vi "XNET Example IP Stack Config - Add Proxy Server.vi"(0 "config in":string, 1 "forwarding destination address":string, 2 "forwarding destination port":u16, 5 "protocol":string(combo)="tcp", 7 "direction":string(combo)="outbound", 9 "listen port":u16, 11 "error in (no error)":errorcluster, 12 "listen address":string, 13 "forwarding source address":string, 14 "forwarding source port":u16) -> (4 "config out":string, 15 "error out":errorcluster)   [LabVIEW 2018]
doc: "This example subVI adds configuration for a single proxy server instance to an existing JSON configuration string for use with XNET IP Stack Create.vi. Configuration parameter definitions:\n\nprotocol: Protocol to use for the proxy server, which can be one of 1) tcp, 2) udp.\n\ndirection: Direction to use for the proxy server, which can be one of 1) outbound, 2) inbound. When using TCP, this specifies the direction of the TCP connection. Once connected, TCP communication is always bidirectional through a single proxy server. When using UDP, this specifies the direction of communication, which is always unidirectional. Use two proxy servers if you require bidirectional UDP communication.\n\nlisten address: The proxy server listens for data on this address. This can be 'any', 'localhost', or a valid IPv4 or IPv6 address using standard IETF syntax. This property is optional; if not provided or if set to an empty string, outbound servers use the default value 'localhost', and inbound servers use the default value 'any'.\n\nlisten port: The proxy server listens for data on this port. Values from 1-65535 identify a valid port number.\n\nforwarding destination address: The proxy server forwards all received data to this address. This can be 'localhost' or a valid IPv4 or IPv6 address using standard IETF syntax.\n\nforwarding destination port: The proxy server forwards all received data to this port. Values from 1-65535 identify a valid port number.\n\nforwarding source address: The proxy server forwards all data using this source address. This can be 'any', 'localhost', or a valid IPv4 or IPv6 address using standard IETF syntax. This property is optional; if not provided or if set to an empty string, the default value 'any' is used.\n\nforwarding source port: The proxy server forwards all data using this source port. Values from 0-65535 identify a valid port number. This property is optional; if not provided, the default value 0 is used, which assigns a randomly-selected port.\n\nYou can re-use this subVI in one of two ways: a) copy the subVI from the example diagram to your VI diagram, which re-uses the subVI unchanged (located in the XNET library), or b) use Save As to create a copy of the subVI in your application folder, and change as needed."
uses:
  XNET Example IP Stack Config - Stack.ctl
  XNET Example IP Stack Config - XNET Interface.ctl
  XNET Example IP Stack Config - MAC.ctl
  XNET Example IP Stack Config - VLAN.ctl
  XNET Example IP Stack Config - Static Address.ctl
  XNET Example IP Stack Config - Static IPv6 Address.ctl
  XNET Example IP Stack Config - Proxy Server.ctl
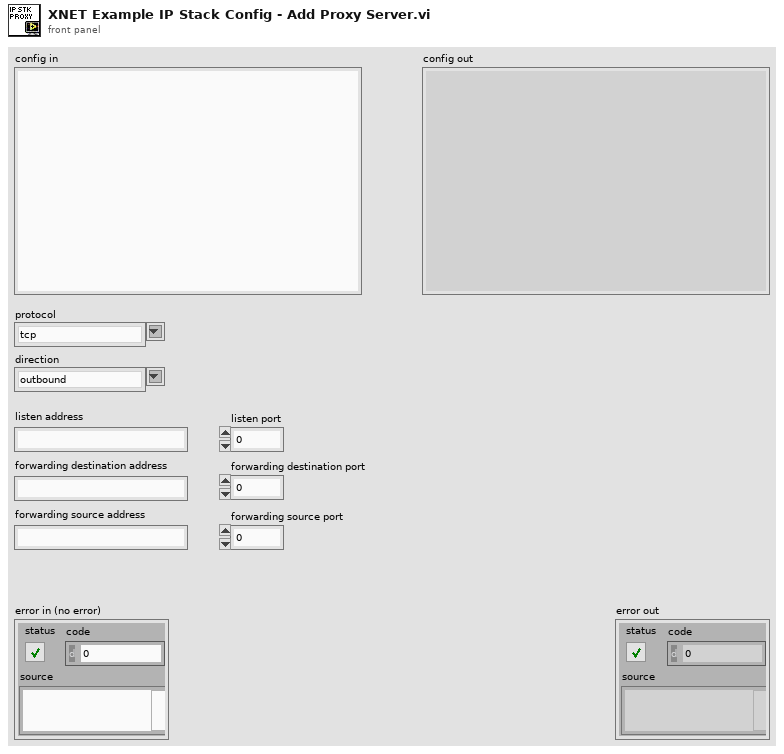
[diagram p1: front panel]
types:
  T1 = typedef "XNET Example IP Stack Config - Proxy Server.ctl" = cluster{"protocol":string, "direction":string, "listenAddress":string, "listenPort":u16, "forwardingDestinationAddress":string, "forwardingDestinationPort":u16, "forwardingSourceAddress":string, "forwardingSourcePort":u16}
  T2 = typedef "XNET Example IP Stack Config - Stack.ctl" = cluster{"schema":string, "xnetInterfaces":T3[], "proxyServers":T1[]}
  T3 = typedef "XNET Example IP Stack Config - XNET Interface.ctl" = cluster{"name":string, "MACs":T4[]}
  T4 = typedef "XNET Example IP Stack Config - MAC.ctl" = cluster{"address":string, "VLANs":T5[]}
  T5 = typedef "XNET Example IP Stack Config - VLAN.ctl" = cluster{"name":string, "isTagged":bool, "id":u16, "IPv4":cluster{"mode":string, "staticAddresses":T6[]}, "IPv6":cluster{"mode":string, "staticAddresses":T7[]}}
  T6 = typedef "XNET Example IP Stack Config - Static Address.ctl" = cluster{"address":string, "subnetMask":string}
  T7 = typedef "XNET Example IP Stack Config - Static IPv6 Address.ctl" = cluster{"address":string}
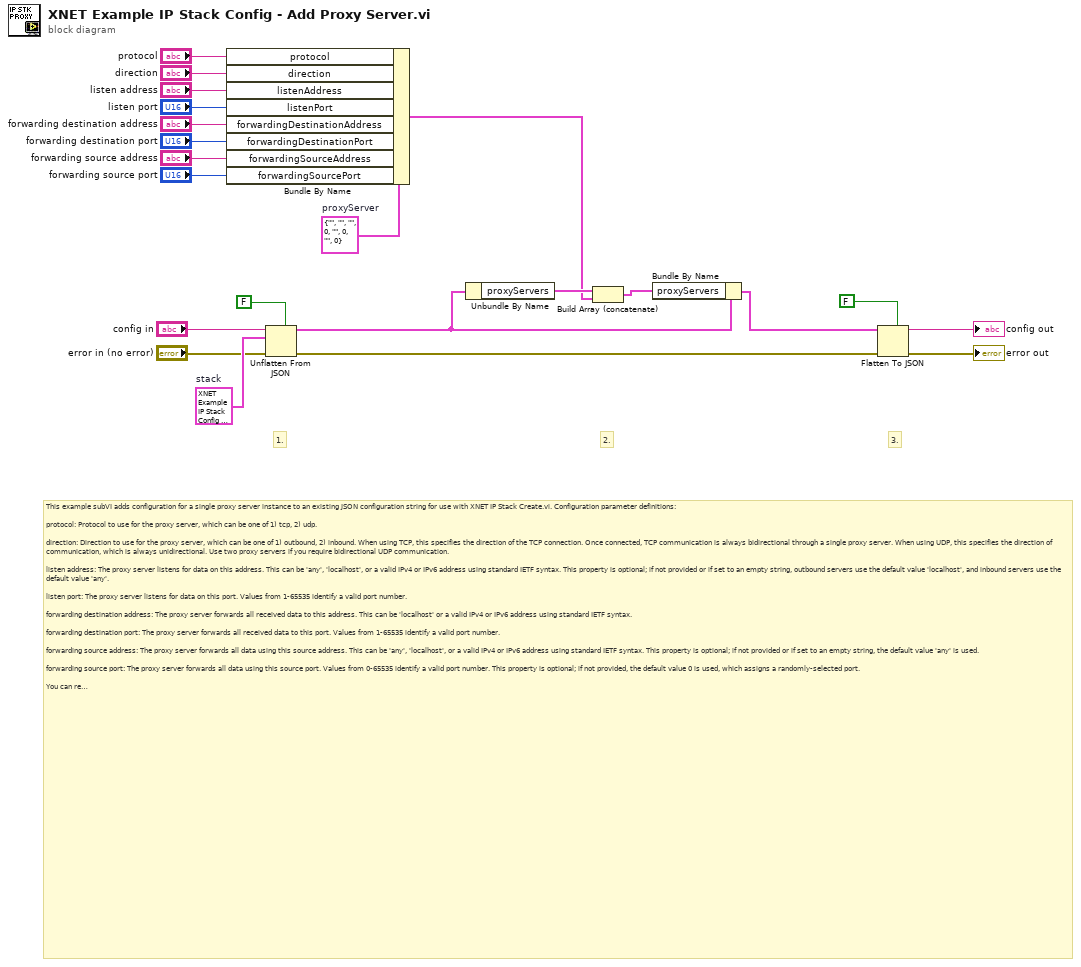
[diagram p0: block diagram]
diagram:
  w16 = T1 {"protocol"="", "direction"="", "listenAddress"="", "listenPort"=0, "forwardingDestinationAddress"="", "forwardingDestinationPort"=0, "forwardingSourceAddress"="", "forwardingSourcePort"=0}  # proxyServer
  w18 = T2 {"schema"="", "xnetInterfaces"=[{"name"="", "MACs"=[{"address"="", "VLANs"=[{"name"="", "isTagged"=FALSE, "id"=0, "IPv4"={"mode"="static", "staticAddresses"=[]}, "IPv6"={"mode"="", "staticAddresses"=[]}}]}]}], "proxyServers"=[]}  # stack
  # "3."
  # "2."
  # "1."
  # "This example subVI adds configuration for a single proxy server instance to an existing JSON configuration string for use with XNET IP Stack Create.vi. Configuration parameter definitions:\n\nprotocol: Protocol to use for the proxy server, which can be one of 1) tcp, 2) udp.\n\ndirection: Direction to use for the proxy server, which can be one of 1) outbound, 2) inbound. When using TCP, this specifies the direction of the TCP connection. Once connected, TCP communication is always bidirectional through a single proxy server. When using UDP, this specifies the direction of communication, which is always unidirectional. Use two proxy servers if you require bidirectional UDP communication.\n\nlisten address: The proxy server listens for data on this address. This can be 'any', 'localhost', or a valid IPv4 or IPv6 address using standard IETF syntax. This property is optional; if not provided or if set to an empty string, outbound servers use the default value 'localhost', and inbound servers use the default value 'any'.\n\nlisten port: The proxy server listens for data on this port. Values from 1-65535 identify a valid port number.\n\nforwarding destination address: The proxy server forwards all received data to this address. This can be 'localhost' or a valid IPv4 or IPv6 address using standard IETF syntax.\n\nforwarding destination port: The proxy server forwards all received data to this port. Values from 1-65535 identify a valid port number.\n\nforwarding source address: The proxy server forwards all data using this source address. This can be 'any', 'localhost', or a valid IPv4 or IPv6 address using standard IETF syntax. This property is optional; if not provided or if set to an empty string, the default value 'any' is used.\n\nforwarding source port: The proxy server forwards all data using this source port. Values from 0-65535 identify a valid port number. This property is optional; if not provided, the default value 0 is used, which assigns a randomly-selected port.\n\nYou can re-use this subVI in one of two ways: a) copy the subVI from the example diagram to your VI diagram, which re-uses the subVI unchanged (located in the XNET library), or b) use Save As to create a copy of the subVI in your application folder, and change as needed.\n1. Use the LabVIEW Unflatten From JSON VI to generate a stack configuration cluster from the JSON configuration string.\n    Since the XNET IP stack JSON is intended to support non-LabVIEW code, avoid LabVIEW-only extensions.\n2. Form a single proxy server configuration and add it to the stack configuration.\n3. Use the LabVIEW Flatten to JSON VI to generate the string from the arrays and clusters.\n    Since the XNET IP stack JSON is intended to support non-LabVIEW code, avoid LabVIEW-only extensions."
  n1 = Bundle By Name(cluster=w16, "protocol"="protocol", "direction"="direction", "listenAddress"="listen address", "listenPort"="listen port", "forwardingDestinationAddress"="forwarding destination address", "forwardingDestinationPort"="forwarding destination port", "forwardingSourceAddress"="forwarding source address", "forwardingSourcePort"="forwarding source port") -> (w5:T1)
  n2 = Unflatten From JSON(enable LabVIEW extensions? (T)=FALSE, JSON string="config in", type and defaults=w18, error in (no error)="error in (no error)") -> (value=w8:T2, error out=w3:errorcluster)  [unwired: 3 in]
  n3 = Unbundle By Name(w8) -> ("proxyServers"=w7:T1[])
  n4 = Build Array (concatenate)(w7, w5) -> (w6:T1[])
  n5 = Bundle By Name(cluster=w8, "proxyServers"=w6) -> (w4:T2)
  n6 = Flatten To JSON(enable LabVIEW extensions? (T)=FALSE, anything=w4, error in (no error)=w3) -> (JSON string=→"config out":string, 11:→"error out":errorcluster)
